vi "Decimal to ASCII.vi"(5 "Decimal Number":u8=84) -> (0 "ASCII Character":string="T", 1 "Hex Number":u8=84 format="%.0x", 2 "Decimal String":string="84")   [LabVIEW 2014]
doc: "The control above is a U8 number that is represented as a decimal.\nThis VI will run continuously and each time the calculate button is pressed, the hexadecimal equivalent of that number is calculated, as well as a string containing that number in normal display mode\nand the ASCII character equivalent of that decimal number in code display mode."
panel:
  # "This VI continuously converts the decimal number to its hexadecimal equivalent, creates a string containing that number in normal display mode, and displays the ASCII character equivalent of the decimal number in code display mode.  \n\nInstructions to execute the VI:\n1. Run the VI\n2. Enter the decimal number to be converted\n3. Click on Convert button"
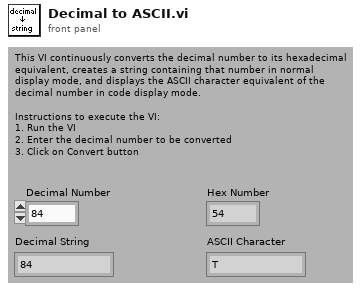
[diagram p1: front panel]
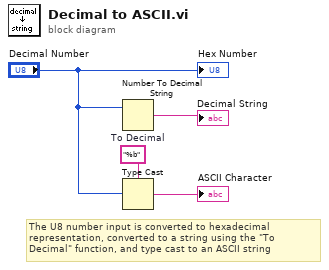
[diagram p0: block diagram]
diagram:
  # "The U8 number input is converted to hexadecimal representation, converted to a string using the \"To Decimal\" function, and type cast to an ASCII string"
  n1 = Number To Decimal String "To Decimal"(number="Decimal Number") -> (decimal integer string=→"Decimal String":string)  [unwired: 1 in]
  n2 = Type Cast(type="%b", x="Decimal Number") -> (*(type *) &x=→"ASCII Character":string)
  "Hex Number" <- "Decimal Number"
